vi "remove group meta data.vi"(8 "error in (no error)":errorcluster, 9 "TDMS datalogger configuration in":refnum<class "TDMS datalogger configuration.lvclass">, 10 "group tag":string, 11 "tree reference":refnum<vi>) -> (0 "error out":errorcluster, 1 "TDMS datalogger configuration out":refnum<class "TDMS datalogger configuration.lvclass">, 3 "tree reference out":refnum<vi>)   [LabVIEW 2015, in "TDMS datalogger editor node.lvclass"]
uses:
  TDMS datalogger editor node.lvclass
  module/configuration/TDMS datalogger configuration.lvclass
  <vilib>/NI/Tag Bus/tag/tag descriptor.lvclass/tag descriptor.ctl
  <vilib>/NI/Tag Bus/tag/tag descriptor.lvclass
panel:
  out "metadata 2":string
  out "metadata":string
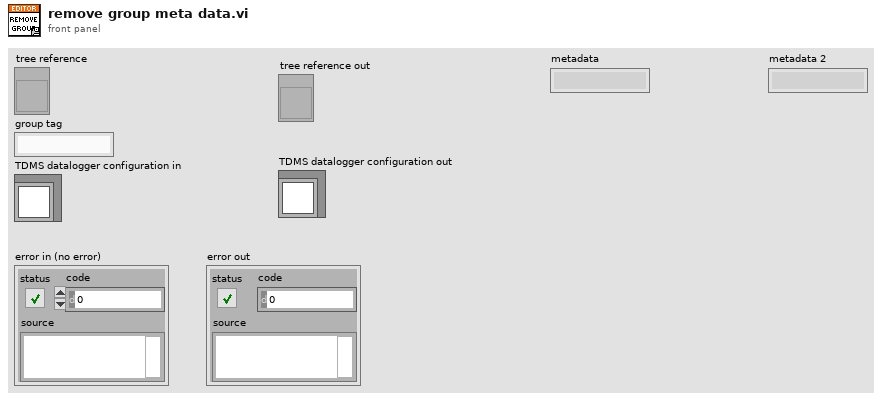
[diagram p1: front panel]
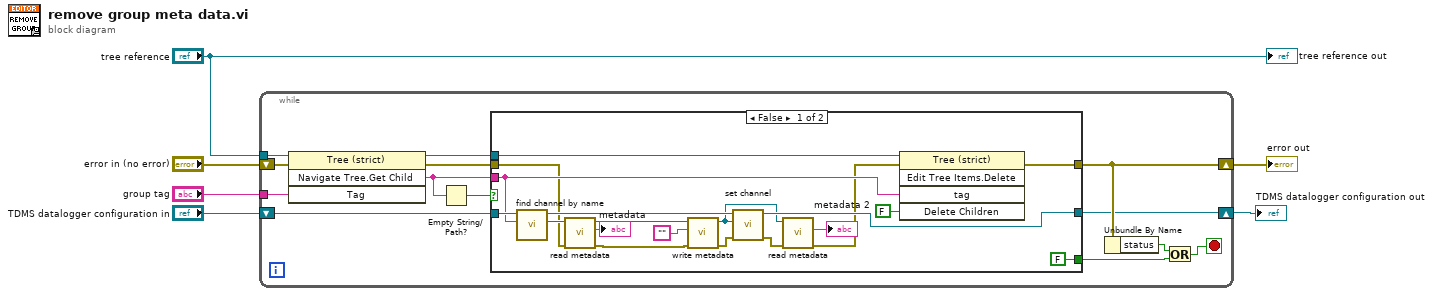
[diagram p0: block diagram]
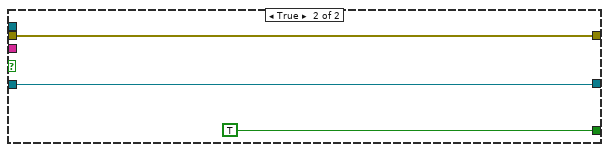
[diagram p2: hidden frame]
diagram:
  n1 = while {
    tunnel: "group tag" -> [w19]
    tunnel: "tree reference" -> [w17]
    shift-right: [w13] -> w2
    shift-left: "error in (no error)" -> [w16]
    shift-right: [w8] -> w1
    shift-left: "TDMS datalogger configuration in" -> [w7]
    stop <- w11 stop-if-true
    n2 = invoke class="Tree (strict)" method="Navigate Tree.Get Child"(reference=w17, error in=w16, "Tag"=w19) -> (reference out=w9:refnum<vi>, error out=w18:errorcluster, "Navigate Tree:Get Child"=w15:string)  [unwired: 1 in, 1 out]
    n3 = Empty String/Path?(string/path=w15) -> (empty?=w14:bool)
    n4 = case shown="False" w14 {
      tunnel: w18 -> [w26 w40]
      tunnel: w15 -> [w34 _]
      tunnel: w7 -> [w37 w39]
      tunnel: [w33 w40] -> w13
      tunnel: [FALSE TRUE] -> w10
      tunnel: w9 -> [w35 _]
      tunnel: [w31 w39] -> w8
      frame False {
        n5 = call "find channel by name.vi"("channel name"=w34, "TDMS datalogger configuration in"=w37) -> ("channel"=w28:refnum<class "TBM channel.lvclass">, "TDMS datalogger configuration out"=w32:refnum<class "TDMS datalogger configuration.lvclass">)  [unwired: 8 in]
        n6 = call <vilib>:"read metadata.vi"("error in"=w26, "system tag in"=w28) -> ("error out"=w24:errorcluster, "metadata"=→"metadata":string, "system tag out"=w27:refnum<class "TBM channel.lvclass">)  [unwired: 7 in]
        n7 = call <vilib>:"write metadata.vi"("error in"=w24, "metadata"="", "system tag in"=w27) -> ("error out"=w30:errorcluster, "system tag out"=w20:refnum<class "TBM channel.lvclass">)  [unwired: 7 in]
        n8 = call "set channel.vi"("error in"=w30, "TBM channel in"=w20, "TDMS datalogger configuration in"=w32) -> ("error out"=w23:errorcluster, "TDMS datalogger configuration out"=w31:refnum<class "TDMS datalogger configuration.lvclass">)  [unwired: 7 in]
        n9 = call <vilib>:"read metadata.vi"("error in"=w23, "system tag in"=w20) -> ("error out"=w22:errorcluster, "metadata"=→"metadata 2":string)  [unwired: 7 in, 1 out]
        n10 = invoke class="Tree (strict)" method="Edit Tree Items.Delete"(reference=w35, error in=w22, "tag"=w34, "Delete Children"=FALSE ("Delete Children?")) -> (error out=w33:errorcluster)  [unwired: 1 in, 4 out]
      }
      frame True {
      }
    }
    n11 = Unbundle By Name(w13) -> ("status"=w12:bool)
    n12 = Or(x=w12, y=w10) -> (x .or. y?=w11:bool)
  }
  "error out" <- w2
  "TDMS datalogger configuration out" <- w1
  "tree reference out" <- "tree reference"
